vi "Create TCP Master.vi"(4 "write operation timeout":i32=1000, 6 "read operation timeout":i32=1000, 8 "error in":errorcluster, 9 "connect timeout ms":i32=10000, 10 "port (502)":u16=502, 11 "address":string) -> (0 "error out":errorcluster, 3 "TCP master instance":refnum<class "Modbus Master.lvclass">)   [LabVIEW 2021, in "API Main.lvlib"]
doc: "Creates a standard TCP master using an IP transmission data unit. This instance looks for a slave at the <B>address</B> and <B>port</B> specified."
uses:
  API Main.lvlib
  Network Protocol/Network Master/TCP/TCP Master.lvclass
  Transmission Data Unit/IP/IP Data Unit.lvclass
  Master Function Definition/Master Function Definition.lvclass
  Transmission Data Unit/Transmission Data Unit.lvclass
  Network Protocol/Network Master/Network Master.lvclass
  C:/my_projects/projects/Algorithms/Labview/21/Modbus_v121c/Transmission Data Unit/Transmission Data Unit.lvclass
  C:/my_projects/projects/Algorithms/Labview/21/Modbus_v121c/Transmission Data Unit/IP/IP Data Unit.lvclass
  Master/Modbus Master.lvclass
  C:/my_projects/projects/Algorithms/Labview/21/Modbus_v121c/Network Protocol/Network Master/Network Master.lvclass
  C:/my_projects/projects/Algorithms/Labview/21/Modbus_v121c/Network Protocol/Network Protocol.lvclass
  C:/my_projects/projects/Algorithms/Labview/21/Modbus_v121c/Network Protocol/Network Master/TCP/TCP Master.lvclass
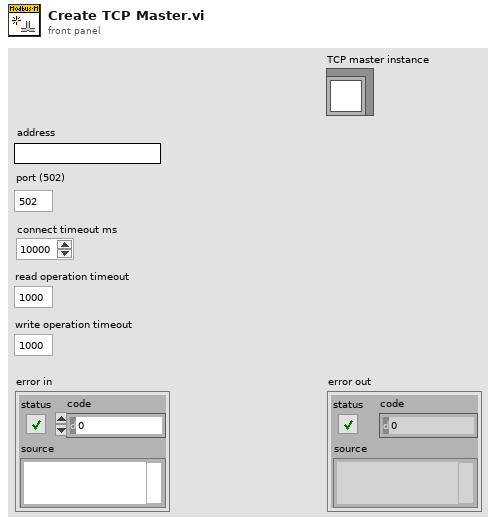
[diagram p1: front panel]
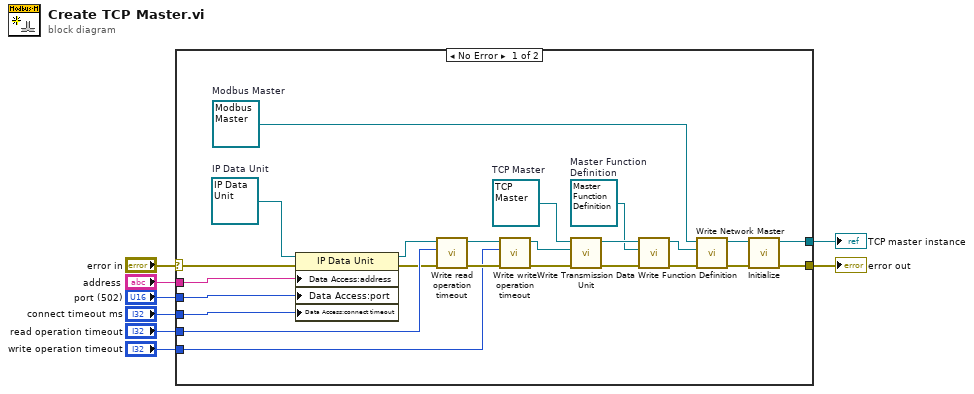
[diagram p0: block diagram]
diagram:
  n1 = case shown="No Error" "error in" {
    selector: "error in" -> [w11 w33]
    tunnel: "address" -> [w32 _]
    tunnel: "port (502)" -> [w31 _]
    tunnel: [w30 w33] -> w1
    tunnel: [w29 _] -> w2
    tunnel: "read operation timeout" -> [w26 _]
    tunnel: "write operation timeout" -> [w25 _]
    tunnel: "connect timeout ms" -> [w24 _]
    frame No Error {
      w21 = refnum<class "Modbus Master.lvclass"> refnum  # Modbus Master
      w23 = refnum<class "IP Data Unit.lvclass"> refnum  # IP Data Unit
      w12 = refnum<class "Master Function Definition.lvclass"> refnum  # Master Function Definition
      w22 = refnum<class "TCP Master.lvclass"> refnum  # TCP Master
      n2 = property class="IP Data Unit"(reference=w23, error in=w11, "Data Access:address"=w32, "Data Access:port"=w31, "Data Access:connect timeout"=w24) -> (reference out=w10:refnum<class "IP Data Unit.lvclass">, error out=w9:errorcluster)
      n3 = call "Write read operation timeout.vi"("error in (no error)"=w9, "read operation timeout"=w26, "transmission data unit in"=w10) -> ("error out"=w27:errorcluster, "transmission data unit out"=w28:refnum<class "IP Data Unit.lvclass">)  [unwired: 7 in]
      n4 = call "Write write operation timeout.vi"("error in (no error)"=w27, "write operation timeout"=w25, "transmission data unit in"=w28) -> ("error out"=w20:errorcluster, "transmission data unit out"=w19:refnum<class "IP Data Unit.lvclass">)  [unwired: 7 in]
      n5 = call "Write Transmission Data Unit.vi"("error in (no error)"=w20, "Transmission Data Unit"=w19, "Network Master in"=w22) -> ("error out"=w14:errorcluster, "Network Master out"=w16:refnum<class "TCP Master.lvclass">)  [unwired: 7 in]
      n6 = call "Write Function Definition.vi"("error in"=w14, "master function definition"=w12, "Modbus master in"=w16) -> ("error out"=w13:errorcluster, "Modbus master out"=w15:refnum<class "TCP Master.lvclass">)  [unwired: 7 in]
      n7 = call "Write Network Master.vi"("error in"=w13, "Network Master"=w15, "Modbus master in"=w21) -> ("error out"=w17:errorcluster, "Modbus master out"=w18:refnum<class "Modbus Master.lvclass">)  [unwired: 7 in]
      n8 = call-dynamic "Initialize.vi"("error in (no error)"=w17, "Modbus master in"=w18) -> ("error out"=w30:errorcluster, "Modbus master out"=w29:refnum<class "Modbus Master.lvclass">)  [unwired: 8 in]
    }
    frame Error {
    }
  }
  "error out" <- w1
  "TCP master instance" <- w2
